vi "Init Main Panels.vi"(8 "error in (no error)":errorcluster, 11 "picoG in":refnum<class "picoG.lvclass">) -> (0 "error out":errorcluster, 3 "picoG out":refnum<class "picoG.lvclass">)   [LabVIEW 2020, in "PicoG-App.lvlib" / "picoG.lvclass"]
uses:
  picoG.lvclass
  GettingStarted/GettingStarted.lvclass
  C:/Program Files (x86)/National Instruments/LabVIEW 2020/vi.lib/IlluminatedG/IG OOPanel/OOPanel/Panel/Panel.lvclass
  AppDetailPanel/AppDetailPanel.lvclass
  PlatformConfigPanel/PlatformConfigPanel.lvclass
  DeviceDetailPanel/DeviceDetailPanel.lvclass
  picoG.lvclass/picoG.ctl
  <vilib>/IlluminatedG/IG OOPanel/OOPanel/Manager/Manager.lvclass
  C:/dev/picoG/PicoG/PicoG-App/GettingStarted/GettingStarted.lvclass
  C:/dev/picoG/PicoG/PicoG-App/PlatformConfigPanel/PlatformConfigPanel.lvclass
  C:/dev/picoG/PicoG/PicoG-App/AppDetailPanel/AppDetailPanel.lvclass
  C:/dev/picoG/PicoG/PicoG-App/DeviceDetailPanel/DeviceDetailPanel.lvclass
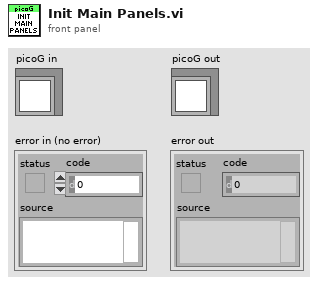
[diagram p1: front panel]
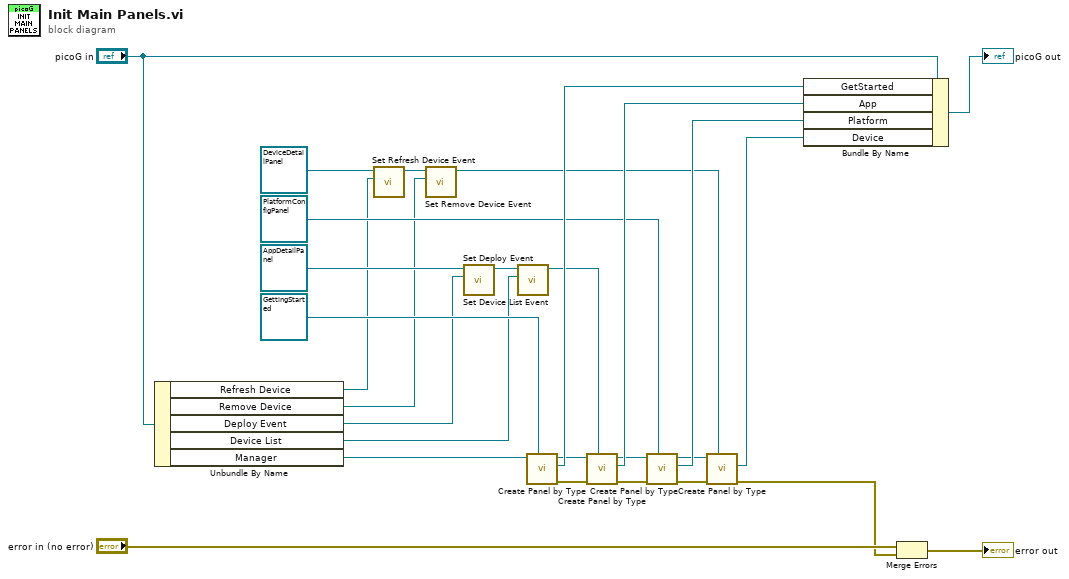
[diagram p0: block diagram]
diagram:
  n1 = Unbundle By Name("picoG in") -> ("Refresh Device"=w1:refnum<user-event>, "Remove Device"=w5:refnum<user-event>, "Deploy Event"=w6:refnum<user-event>, "Device List"=w10:refnum<user-event>, "Manager"=w25:refnum<class "Manager.lvclass">)
  n2 = call "Set Refresh Device Event.vi"("Refresh Device"=w1, "DeviceDetailPanel in"=refnum<class "DeviceDetailPanel.lvclass"> refnum ("PicoG-App.lvlib:DeviceDetailPanel.lvclass")) -> ("DeviceDetailPanel out"=w3:refnum<class "DeviceDetailPanel.lvclass">)  [unwired: 8 in, 1 out]
  n3 = call "Set Remove Device Event.vi"("Remove Device"=w5, "DeviceDetailPanel in"=w3) -> ("DeviceDetailPanel out"=w4:refnum<class "DeviceDetailPanel.lvclass">)  [unwired: 8 in, 1 out]
  n4 = call "Set Deploy Event.vi"("Deploy Event"=w6, "AppDetailPanel in"=refnum<class "AppDetailPanel.lvclass"> refnum ("PicoG-App.lvlib:AppDetailPanel.lvclass")) -> ("AppDetailPanel out"=w7:refnum<class "AppDetailPanel.lvclass">)  [unwired: 8 in, 1 out]
  n5 = call "Set Device List Event.vi"("Device List"=w10, "AppDetailPanel in"=w7) -> ("AppDetailPanel out"=w9:refnum<class "AppDetailPanel.lvclass">)  [unwired: 8 in, 1 out]
  n6 = call <vilib>:"Create Panel by Type.vi"("Panel Type"=refnum<class "GettingStarted.lvclass"> refnum ("PicoG-App.lvlib:GettingStarted.lvclass"), "Manager in"=w25) -> ("error out"=w20:errorcluster, "Panel"=w23:refnum<class "GettingStarted.lvclass">, "Manager out"=w22:refnum<class "Manager.lvclass">)  [unwired: 7 in]
  n7 = call <vilib>:"Create Panel by Type.vi"("Panel Type"=w9, "error in (no error)"=w20, "Manager in"=w22) -> ("error out"=w18:errorcluster, "Panel"=w21:refnum<class "AppDetailPanel.lvclass">, "Manager out"=w17:refnum<class "Manager.lvclass">)  [unwired: 6 in]
  n8 = call <vilib>:"Create Panel by Type.vi"("Panel Type"=refnum<class "PlatformConfigPanel.lvclass"> refnum ("PicoG-App.lvlib:PlatformConfigPanel.lvclass"), "error in (no error)"=w18, "Manager in"=w17) -> ("error out"=w13:errorcluster, "Panel"=w15:refnum<class "PlatformConfigPanel.lvclass">, "Manager out"=w14:refnum<class "Manager.lvclass">)  [unwired: 6 in]
  n9 = call <vilib>:"Create Panel by Type.vi"("Panel Type"=w4, "error in (no error)"=w13, "Manager in"=w14) -> ("error out"=w12:errorcluster, "Panel"=w11:refnum<class "DeviceDetailPanel.lvclass">)  [unwired: 6 in, 1 out]
  n10 = Bundle By Name(cluster="picoG in", "GetStarted"=w23, "App"=w21, "Platform"=w15, "Device"=w11) -> (→"picoG out":refnum<class "picoG.lvclass">)
  n11 = Merge Errors("error in (no error)", w12) -> (→"error out":errorcluster)
